vi "TCP Server Core - VI Tree.vi"() -> ()   [LabVIEW 2020, in "JKI TCP Server.lvclass"]
uses:
  JKI TCP Server.lvclass
  JKI TCP Server.lvclass/JKI TCP Server.ctl
  _Data Structures/TCP Server Connection Process Data Cluster.ctl
panel:
  in  "Connection Data":T1
  # "OpenGOOP Core VI Tree\nSee Diagram"
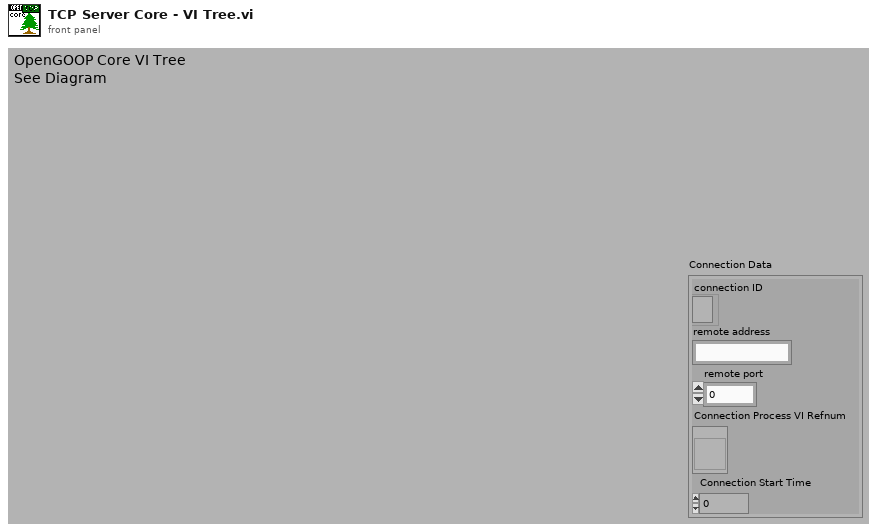
[diagram p1: front panel]
types:
  T1 = typedef "JKI TCP Server.lvclass/TCP Server Connection Process Data Cluster.ctl" = cluster{"connection ID":refnum<k5>, "remote address":string, "remote port":u16, "Connection Process VI Refnum":refnum<vi>, "Connection Start Time":u32}
  T2 = typedef "JKI TCP Server.lvclass/TCP Server Data.ctl" = cluster{"Listener Info":T3, "Connection Process VI RefNums":refnum<vi>[], "dup connection IDs (for quick search)":refnum<k5>[], "Connections":T4[], "Connection Handler VI Path":path, "Handler Is Reentrant?":bool, "TCP Handler Instance RefNums":T5[], "TCP Handler VI RefNum":T5, "No. Connections":u32, "Max Connections":u32, "server start time":u32, "Additional Data":variant}
  T3 = typedef "JKI TCP Server.lvclass/TCP Server Listener Info Cluster.ctl" = cluster{"listener ID":refnum<k5>, "net address":u32, "port":u16, "Listener Process VI Refnum":refnum<vi>}
  T4 = typedef "JKI TCP Server.lvclass/TCP Server Connection Info Cluster.ctl" = cluster{"connection ID":refnum<k5>, "Remote Address":string, "remote port":u16, "connection start time":u32}
  T5 = typedef "JKI TCP Server.lvclass/TCP Server Handler RefNum.ctl" = refnum<vi>
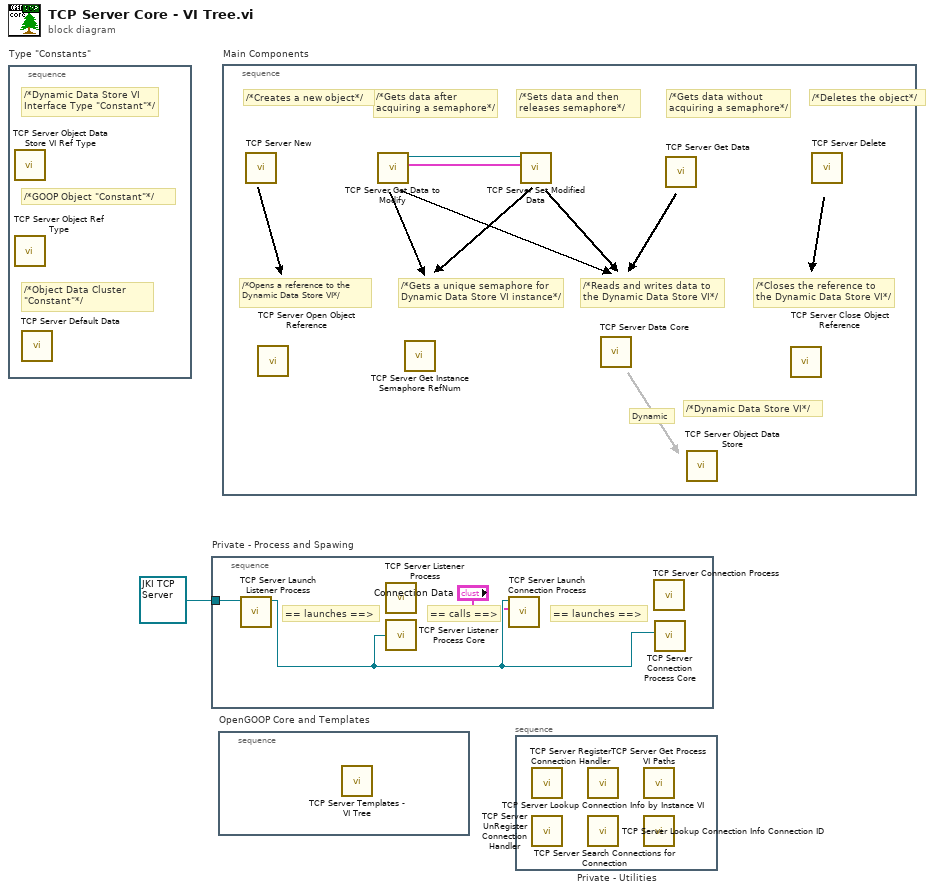
[diagram p0: block diagram]
diagram:
  n1 = stacked-sequence "Type \"Constants\"" {
    frame #0 {
      # "/*Dynamic Data Store VI Interface Type \"Constant\"*/"
      # "/*GOOP Object \"Constant\"*/"
      # "/*Object Data Cluster \"Constant\"*/"
      n2 = call "TCP Server Object Data Store VI Ref Type.vi"() -> ()  [unwired: 5 in, 1 out]
      n3 = call "TCP Server Object Ref Type.vi"() -> ()  [unwired: 5 in, 1 out]
      n4 = call "TCP Server Default Data.vi"() -> ()  [unwired: 1 out]
    }
  }
  n5 = stacked-sequence "Private - Process and Spawing" {
    tunnel: refnum<class "JKI TCP Server.lvclass"> refnum ("TCP Server") -> [w2]
    frame #0 {
      # "== calls ==>"
      # "== launches ==>"
      # "== launches ==>"
      n6 = call "TCP Server Launch Listener Process.vi"("RefNum"=w2) -> ("dup RefNum"=w4:refnum<class "JKI TCP Server.lvclass">)  [unwired: 9 in, 1 out]
      n7 = call "TCP Server Listener Process.vi"() -> ()  [unwired: 1 in]
      n8 = call "TCP Server Listener Process Core.vi"("TCP Server RefNum"=w4) -> ()
      n9 = call "TCP Server Launch Connection Process.vi"("Connection Data"="Connection Data", "TCP Server RefNum"=w4) -> ()  [unwired: 9 in, 1 out]
      n10 = call "TCP Server Connection Process.vi"() -> ()  [unwired: 1 in]
      n11 = call "TCP Server Connection Process Core.vi"("TCP Server Refnum"=w4) -> ()  [unwired: 11 in]
    }
  }
  n12 = stacked-sequence "OpenGOOP Core and Templates" {
    frame #0 {
      n13 = call "TCP Server Templates - VI Tree.vi"() -> ()  [unwired: 1 in]
    }
  }
  n14 = stacked-sequence "Main Components" {
    frame #0 {
      # "Dynamic"
      # "/*Opens a reference to the Dynamic Data Store VI*/"
      # "/*Reads and writes data to the Dynamic Data Store VI*/"
      # "/*Closes the reference to the Dynamic Data Store VI*/"
      # "/*Dynamic Data Store VI*/"
      # "/*Gets a unique semaphore for Dynamic Data Store VI instance*/"
      # "/*Creates a new object*/"
      # "/*Gets data after acquiring a semaphore*/"
      # "/*Sets data and then releases semaphore*/"
      # "/*Deletes the object*/"
      # "/*Gets data without acquiring a semaphore*/"
      n15 = call "TCP Server New.vi"() -> ()  [unwired: 10 in, 2 out]
      n16 = call "TCP Server Open Object Reference.vi"() -> ()  [unwired: 10 in, 2 out]
      n17 = call "TCP Server Get Data to Modify.vi"() -> ("Data out"=w6:T2, "dup RefNum"=w5:refnum<class "JKI TCP Server.lvclass">)  [unwired: 8 in, 2 out]
      n18 = call "TCP Server Get Instance Semaphore RefNum.vi"() -> ()  [unwired: 9 in, 3 out]
      n19 = call "TCP Server Set Modified Data.vi"("Data in"=w6, "RefNum"=w5) -> ()  [unwired: 8 in, 2 out]
      n20 = call "TCP Server Data Core.vi"() -> ()  [unwired: 9 in, 3 out]
      n21 = call "TCP Server Get Data.vi"() -> ()  [unwired: 9 in, 3 out]
      n22 = call "TCP Server Object Data Store.vi"() -> ()  [unwired: 11 in, 1 out]
      n23 = call "TCP Server Close Object Reference.vi"() -> ()  [unwired: 11 in, 1 out]
      n24 = call "TCP Server Delete.vi"() -> ()  [unwired: 11 in, 1 out]
    }
  }
  n25 = stacked-sequence "Private - Utilities" {
    frame #0 {
      n26 = call "TCP Server Register Connection Handler.vi"() -> ()  [unwired: 9 in, 3 out]
      n27 = call "TCP Server UnRegister Connection Handler.vi"() -> ()  [unwired: 9 in, 3 out]
      n28 = call "TCP Server Lookup Connection Info by Instance VI.vi"() -> ()  [unwired: 6 in, 6 out]
      n29 = call "TCP Server Lookup Connection Info Connection ID.vi"() -> ()  [unwired: 10 in, 2 out]
      n30 = call "TCP Server Get Process VI Paths.vi"() -> ()  [unwired: 1 out]
      n31 = call "TCP Server Search Connections for Connection.vi"() -> ()  [unwired: 3 in, 3 out]
    }
  }
